vi "Read DVR.vi"(8 "error in (no error)":errorcluster, 11 "PAS UI in":refnum<class "PAS UI.lvclass">) -> (0 "error out":errorcluster, 2 "DVR":refnum<data-value>, 3 "PAS UI out":refnum<class "PAS UI.lvclass">)   [LabVIEW 2012, in "PAS UI.lvclass"]
uses:
  PAS UI.lvclass
  Data/cPAS Data.lvclass
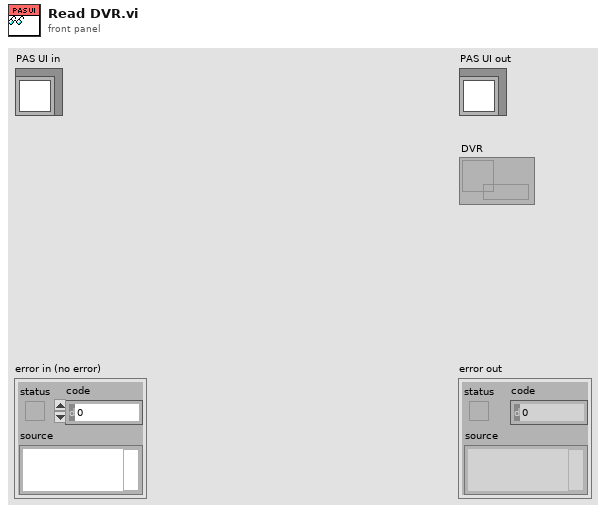
[diagram p1: front panel]
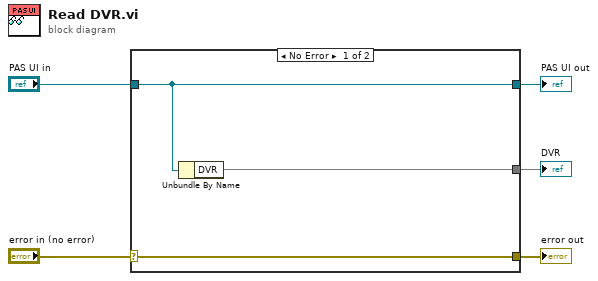
[diagram p0: block diagram]
diagram:
  n1 = case shown="No Error" "error in (no error)" {
    selector: "error in (no error)" -> [w8 w9]
    tunnel: [w8 w9] -> w4
    tunnel: [w7 w10] -> w2
    tunnel: "PAS UI in" -> [w7 w10]
    tunnel: [w6 _] -> w1
    frame No Error {
      n2 = Unbundle By Name(w7) -> ("DVR"=w6)
    }
    frame Error {
    }
  }
  "error out" <- w4
  "PAS UI out" <- w2
  "DVR" <- w1
